vi "PH_DeformableMirror.evt call SetAllChannels.vi"(0 "i ref in":refnum<vi>, 1 "Object":string="N/A", 3 "Voltages":dbl[](array[numeric]), 5 "error in (no error)":errorcluster) -> (14 "i ref out":refnum<vi>, 19 "error out":errorcluster)   [LabVIEW 2014, in "PH_DeformableMirror.lvlib"]
uses:
  PH_DeformableMirror.lvlib
  CS_Core/CSSystem/CoreLib/CoreLib.double array 2 byte array.vi
  CS_Core/CSSystem/CoreLib/CoreLib.lvlib
  CS_Core/BaseProcess/BaseProcess.lvlib
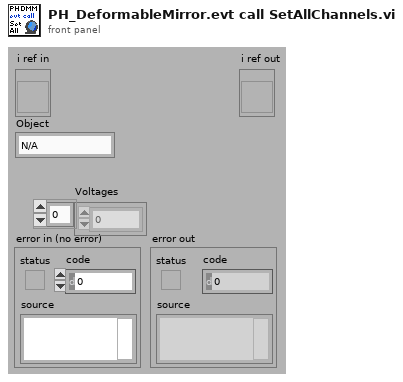
[diagram p1: front panel]
types:
  T1 = typedef "CoreDefs.rawDataType.ctl" = i8[]
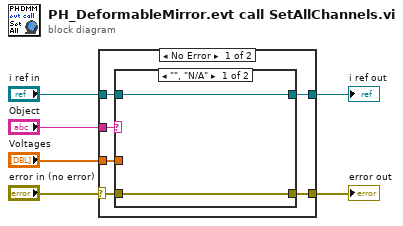
[diagram p0: block diagram]
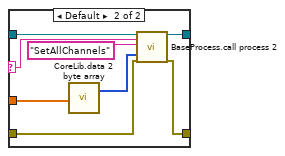
[diagram p2: hidden frame]
diagram:
  n1 = case shown="No Error" "error in (no error)" {
    selector: "error in (no error)" -> [w9 w23]
    tunnel: "i ref in" -> [w12 w24]
    tunnel: [w11 w24] -> w5
    tunnel: [w10 w23] -> w4
    tunnel: "Object" -> [w8 _]
    tunnel: "Voltages" -> [w7 _]
    frame No Error {
      n2 = case shown="\"\", \"N/A\"" w8 {
        selector: w8 -> [_ w18]
        tunnel: w12 -> [w14 w22]
        tunnel: [w14 w21] -> w11
        tunnel: [w13 w20] -> w10
        tunnel: w9 -> [w13 w19]
        tunnel: w7 -> [_ w15]
        frame "", "N/A" {
        }
        frame Default {
          n3 = call-poly "CoreLib.data 2 byte array.vi"("[d64]"=w15) -> ("byteArray out"=w16:T1)  [unwired: 18 in]
          n4 = call "BaseProcess.call process 2.vi"("i ref in"=w22, "Object"=w18, "Selector"="SetAllChannels", "Data"=w16, "error in (no error)"=w19) -> ("i ref out"=w21:refnum<vi>, "error out"=w20:errorcluster)  [unwired: 13 in]
        }
      }
    }
    frame Error {
    }
  }
  "error out" <- w4
  "i ref out" <- w5
